vi "dxf提取直线坐标点.vi"(11 "字符串":string) -> (3 "数组":cluster{i32, i32}[](array[cluster]))   [LabVIEW 2014]
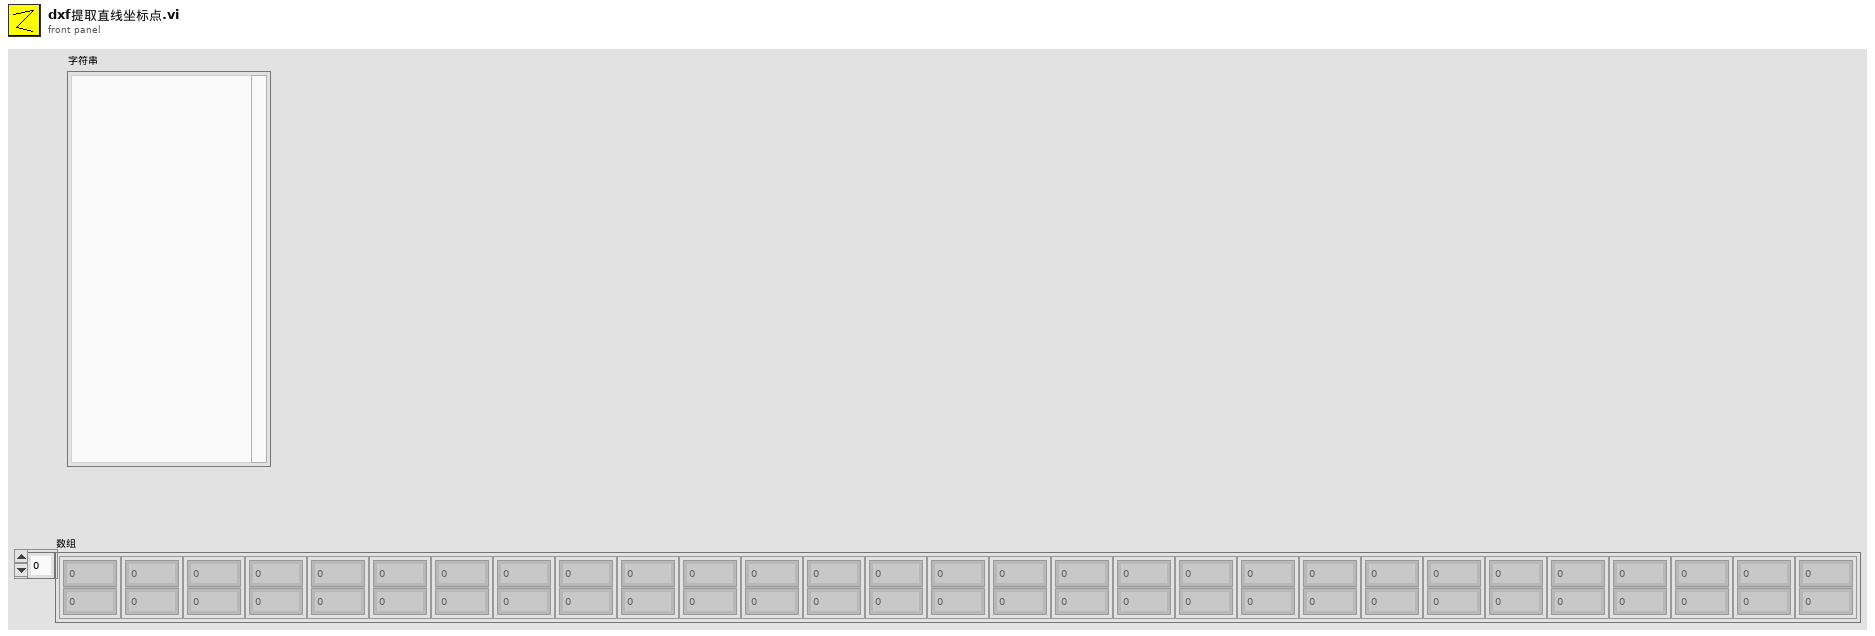
[diagram p1: front panel]
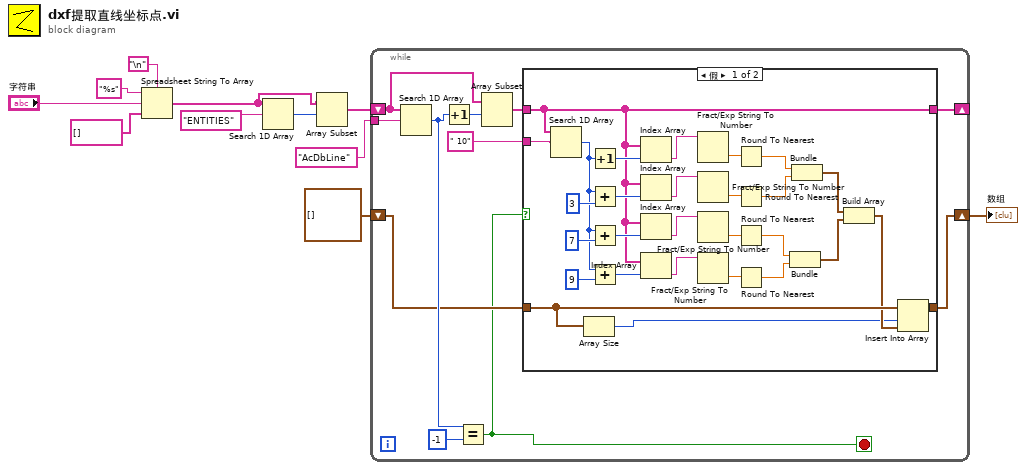
[diagram p0: block diagram]
diagram:
  n1 = Spreadsheet String To Array(delimiter (Tab)="\n", format string="%s" ("格式字符串"), spreadsheet string="字符串", array type (2D Dbl)=string[] [] ("数组类型(2D Dbl)")) -> (array=w5:string[])
  n2 = Search 1D Array(1D array=w5, element="ENTITIES" ("元素")) -> (index of element=w6:i32)  [unwired: 1 in]
  n3 = Array Subset(array=w5, index=w6) -> (w4:string[])  [unwired: 1 in]
  n4 = while {
    tunnel: "AcDbLine" ("元素") -> [w22]
    shift-right: [w13] -> _
    shift-left: w4 -> [w19]
    shift-right: [w16] -> w1
    shift-left: cluster{i32, i32}[] [] -> [w15]
    stop <- w12 stop-if-true
    n5 = Search 1D Array(1D array=w19, element=w22) -> (index of element=w18:i32)  [unwired: 1 in]
    n6 = Increment(x=w18) -> (x+1=w20:i32)
    n7 = Equal?(x=w18, y=-1) -> (x = y?=w12:bool)
    n8 = Array Subset(array=w19, index=w20) -> (w17:string[])  [unwired: 1 in]
    n9 = case shown="假" w12 {
      tunnel: w17 -> [w23 w52]
      tunnel: [w28 w51] -> w16
      tunnel: w15 -> [w27 w51]
      tunnel: " 10" -> [w25 _]
      tunnel: [w23 w52] -> w13
      frame False {
        n10 = Search 1D Array(1D array=w23, element=w25) -> (index of element=w43:i32)  [unwired: 1 in]
        n11 = Array Size(array=w27) -> (size(s)=w24:i32)
        n12 = Increment(x=w43) -> (x+1=w50:i32)
        n13 = Add(x=w43, y=i8 3) -> (x+y=w49:i32)
        n14 = Add(x=w43, y=i8 7) -> (x+y=w48:i32)
        n15 = Add(x=w43, y=i8 9) -> (x+y=w47:i32)
        n16 = Index Array(array=w23, index=w50) -> (element=w42:string)
        n17 = Index Array(array=w23, index=w49) -> (element=w41:string)
        n18 = Index Array(array=w23, index=w48) -> (element=w40:string)
        n19 = Index Array(array=w23, index=w47) -> (element=w39:string)
        n20 = Fract/Exp String To Number(string=w42) -> (number=w38:dbl)  [unwired: 3 in, 1 out]
        n21 = Fract/Exp String To Number(string=w41) -> (number=w37:dbl)  [unwired: 3 in, 1 out]
        n22 = Fract/Exp String To Number(string=w40) -> (number=w36:dbl)  [unwired: 3 in, 1 out]
        n23 = Fract/Exp String To Number(string=w39) -> (number=w35:dbl)  [unwired: 3 in, 1 out]
        n24 = Round To Nearest(number=w38) -> (nearest integer value=w34:dbl)
        n25 = Round To Nearest(number=w37) -> (nearest integer value=w33:dbl)
        n26 = Round To Nearest(number=w36) -> (nearest integer value=w31:dbl)
        n27 = Round To Nearest(number=w35) -> (nearest integer value=w32:dbl)
        n28 = Bundle(w31, w32) -> (w29:cluster{dbl, dbl})  [unwired: 1 in]
        n29 = Bundle(w34, w33) -> (w30:cluster{dbl, dbl})  [unwired: 1 in]
        n30 = Build Array(w30, w29) -> (w26:cluster{dbl, dbl}[])
        n31 = Insert Into Array(array=w27, index=w24, new element=w26) -> (w28:cluster{i32, i32}[])
      }
      frame True {
      }
    }
  }
  "数组" <- w1
